vi "Decimate DFD.vi"(8 "error in (no error)":errorcluster, 10 "output fs[Hz]":dbl=6500.0 format="%#_13g", 11 "Waveforms in":waveform(dbl)[](array[waveform])) -> (0 "error out":errorcluster, 3 "waveforms out":waveform(dbl)[](array[waveform]))   [LabVIEW 2019, in "Instrument.Lockin.lvlib" / "Instrument.DAQ.lvclass"]
uses:
  Instrument.DAQ.lvclass
  <vilib>/addons/Digital Filter Design/_Objects.llb/DFD Multirate Filtering Mode.ctl
  <vilib>/Analysis/2dsp.llb/Decimate (single shot, DBL).vi
  <vilib>/addons/Digital Filter Design/NI_DigFilterLicensed.lvlib
  <vilib>/addons/Digital Filter Design/_Objects.llb/DFD Multirate Filter Specification (Design).ctl
  <vilib>/Analysis/NI_AALPro.lvlib
  <vilib>/measure/NI_MAPro.lvlib
  <vilib>/addons/Digital Filter Design/_Objects.llb/DFD Filter Ripple Specification (Design).ctl
  <vilib>/addons/Digital Filter Design/Multirate.llb/DFD MRate Filtering for Single Block (Wfm NChan).vi
  <vilib>/measure/maresamp.llb/Resample N Waveforms (continuous).vi
  <vilib>/addons/Digital Filter Design/Multirate.llb/DFD NStage MRate Filtering for Single Block (Wfm).vi
  <vilib>/addons/Digital Filter Design/Multirate.llb/DFD NStage MRate Filtering (Wfm).vi
panel:
  out "x != y?":bool
  out "x/y":dbl
  out "Magnitude Response":cluster{"f0":dbl, "df":dbl, "values":dbl[]}[](graph)
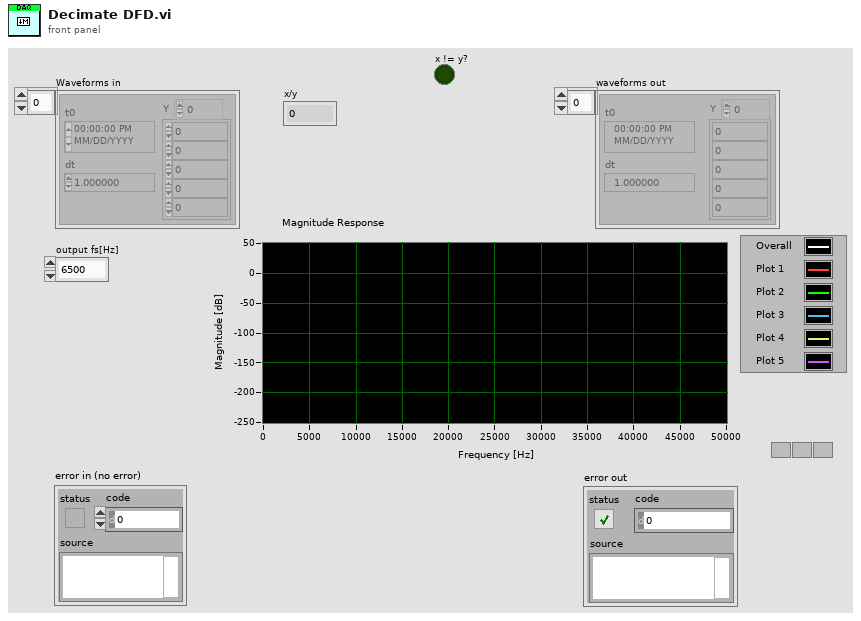
[diagram p1: front panel]
types:
  T1 = typedef "NI_DigFilterLicensed.lvlib/DFD Multirate Filtering Mode.ctl" = u16
  T2 = typedef "NI_DigFilterLicensed.lvlib/DFD Filter Ripple Specification (Design).ctl" = cluster{"passband":dbl, "stopband":dbl, "dB/linear? (T: dB)":bool}
  T3 = typedef "NI_DigFilterLicensed.lvlib/DFD Multirate Filter Specification (Design).ctl" = cluster{"fpass":dbl, "fstop":dbl}
  T4 = typedef "NI_DigFilterLicensed.lvlib/DFD Multirate Filter Obj.ctl" = cluster{"mMRate_Structure":enum16{"CIC", "FIR", "IIR", "Lattice"}, "mMRate_Mode":T5, "mMRate_Factor":i32, "mMRate_FIRParams":cluster{"mMRate_FIR_H":dbl[], "mMRate_FIR_IsNyquist?":bool, "mMRate_FIR_IsSymmetric?":bool}, "mMRate_CICParams":cluster{"mMRate_CIC_#Stage":i32, "mMRate_CIC_Lag":i32, "mMRate_CIC_Type":enum16{"Lowpass", "Highpass"}}, "mMRate_Order":i32, "mMRate_Version":string, "mMRate_Comments":string, "mMRate_RationalFactor":cluster{"mMRate_L":i32, "mMRate_M":i32}, "mMRate_Fs":dbl, "mMRate_Quantized?":bool, "mMRate_QFilterGain":dbl, "mMRate_CoefWl":i16, "mMRate_Scaling":cluster{"mMRate_ScaleByPowerOf2?":bool, "mMRate_ScaleType":T6}, "mMRate_InputWl":i16, "mMRate_OutputWl":i16, "mMRate_OutputMode":T7, "mMRate_MultMode":T8, "mMRate_BitPruning":bool, "mMRate_GainWl":i16, "mMRate_OutputFwl":i16, "mMRate_SumIwl":i16, "mMRate_InputIwl ":i16, "mMRate_SumWl":i16, "mMRate_CoefIwl":i16}
  T5 = typedef "NI_DigFilterLicensed.lvlib/DFD Multirate Mode.ctl" = i16
  T6 = typedef "NI_DigFilterLicensed.lvlib/DFD Coef Norm Type.ctl" = enum16{"No Norm", "Time Domain 1-Norm", "Time Domain 2-Norm", "Time Domain Inf-Norm"}
  T7 = typedef "NI_DigFilterLicensed.lvlib/DFD Round-off Mode.ctl" = enum16{"Nearest", "Truncation"}
  T8 = typedef "NI_DigFilterLicensed.lvlib/DFD FXP MRate Multiply Mode.ctl" = enum16{"Truncated", "Full"}
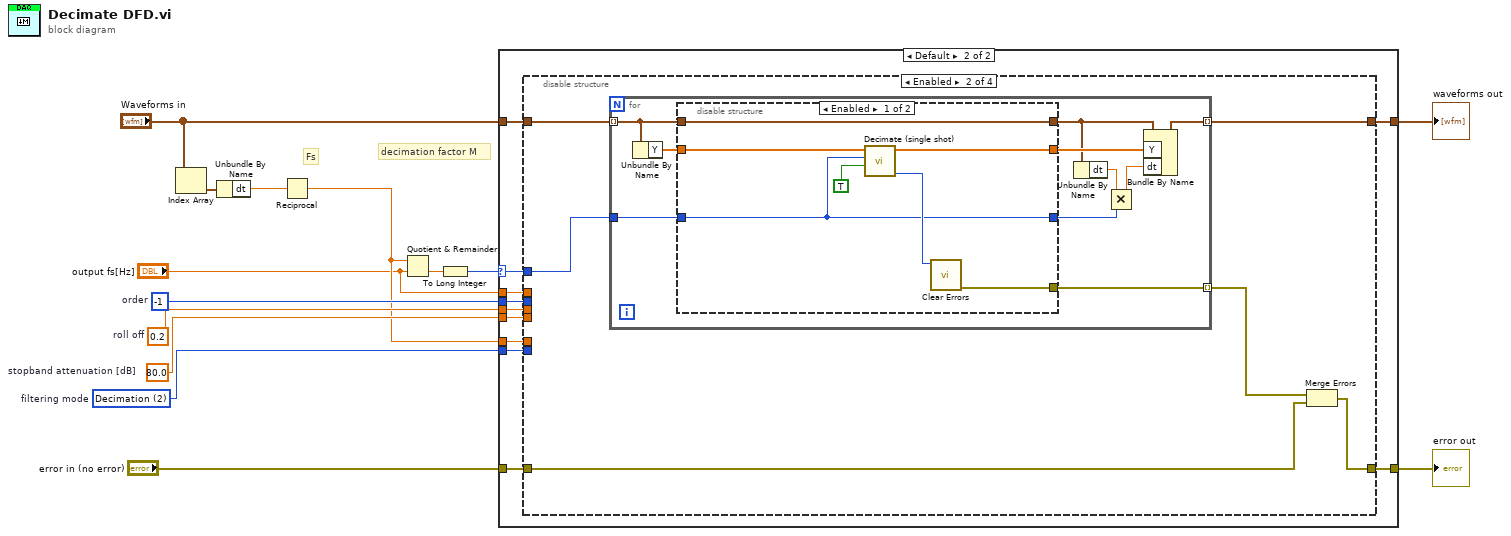
[diagram p0: block diagram]
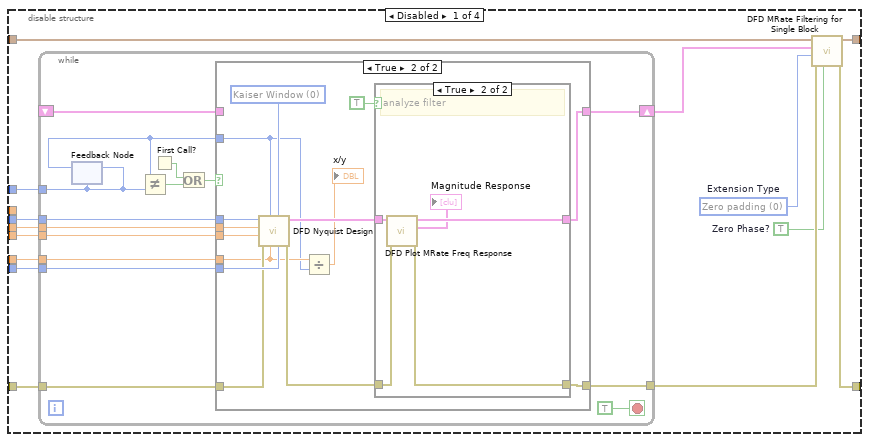
[diagram p3: hidden frame]
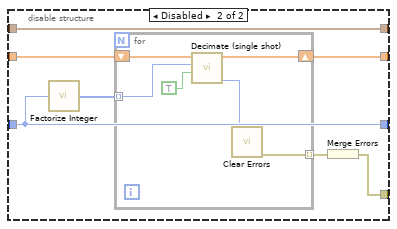
[diagram p6: hidden frame]
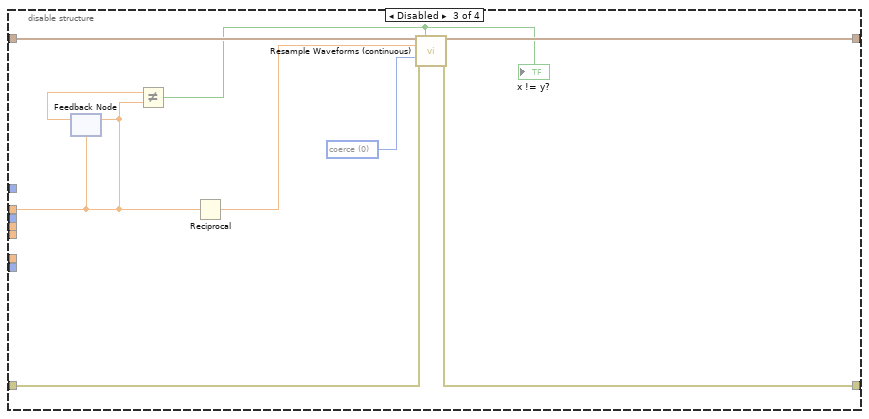
[diagram p7: hidden frame]
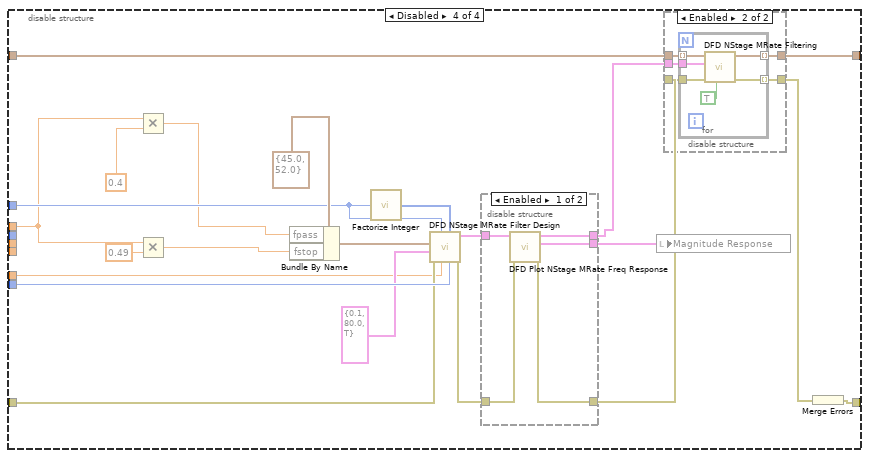
[diagram p8: hidden frame]
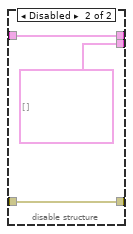
[diagram p9: hidden frame]
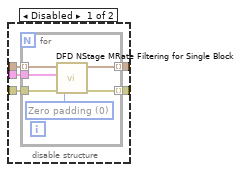
[diagram p10: hidden frame]
diagram:
  w13 = -1  # order
  w10 = 80.0  # stopband attenuation [dB]
  w11 = T1 2 items=["No Rate Change", "Interpolation", "Decimation"]  # filtering mode
  w14 = 0.2  # roll off
  # "Fs"
  # "decimation factor M"
  n1 = Index Array(array="Waveforms in") -> (element=w7:waveform(dbl))  [unwired: 1 in]
  n2 = Unbundle By Name(w7) -> ("dt"=w3:dbl)
  n3 = Reciprocal(x=w3) -> (1/x=w2:dbl)
  n4 = Quotient & Remainder(x=w2, y="output fs[Hz]") -> (floor(x/y)=w12:dbl)  [unwired: 1 out]
  n5 = To Long Integer(number=w12) -> (32bit integer=w8:i32)
  n6 = case shown="Default" w8 {
    selector: w8 -> [_ w21]
    tunnel: w14 -> [_ w27]
    tunnel: w11 -> [_ w26]
    tunnel: w10 -> [_ w25]
    tunnel: w13 -> [_ w24]
    tunnel: "Waveforms in" -> [w16 w20]
    tunnel: [w16 w23] -> w9
    tunnel: w2 -> [_ w22]
    tunnel: "output fs[Hz]" -> [_ w19]
    tunnel: [w15 w18] -> w5
    tunnel: "error in (no error)" -> [w15 w17]
    frame 0, 1 {
    }
    frame Default {
      n7 = disable-structure shown="Enabled" {
        disable-tunnel: w27 -> [w41 _ _ _]
        disable-tunnel: w26 -> [w40 _ _ w145]
        disable-tunnel: w25 -> [w39 _ _ _]
        disable-tunnel: w24 -> [w38 _ _ _]
        disable-tunnel: [w37 w81 w123 w144] -> w23
        disable-tunnel: w22 -> [w36 _ _ w125]
        disable-tunnel: w20 -> [w33 w82 w124 w128]
        disable-tunnel: w21 -> [w32 w85 _ w136]
        disable-tunnel: w19 -> [_ _ w118 w133]
        disable-tunnel: [w31 w83 w121 w137] -> w18
        disable-tunnel: w17 -> [w28 w84 w122 w140]
        frame Disabled {
          w29 = TRUE  # Zero Phase?
          w30 = u16 0 items=["Zero padding", "Symmetric", "Periodic"]  # Extension Type
          n8 = while {
            tunnel: w41 -> [w56]
            tunnel: w40 -> [w55]
            tunnel: w39 -> [w54]
            tunnel: w38 -> [w53]
            tunnel: w36 -> [w52]
            tunnel: [w50] -> w34
            shift-right: [w51] -> w35
            shift-left: _ -> [w48]
            tunnel: w32 -> [w43]
            tunnel: w28 -> [w44]
            stop <- TRUE stop-if-true
            n9 = feedback #1(w43) -> (w42:i32)
            n10 = feedback-in #1(w43) -> ()
            n11 = Not Equal?(x=w42, y=w43) -> (x != y?=w46:bool)
            n12 = First Call?() -> (First Call?: T/F=w47:bool)
            n13 = Or(x=w47, y=w46) -> (x .or. y?=w45:bool)
            n14 = case shown="True" w45 {
              tunnel: w56 -> [_ w72]
              tunnel: w55 -> [_ w71]
              tunnel: w54 -> [_ w70]
              tunnel: w53 -> [_ w69]
              tunnel: w52 -> [_ w61]
              tunnel: [w57 w66] -> w51
              tunnel: [w58 w65] -> w50
              tunnel: w48 -> [w57 _]
              tunnel: w42 -> [_ w60]
              tunnel: w44 -> [w58 w62]
              frame False {
              }
              frame True {
                w68 = u16 0 items=["Kaiser Window", "Dolph-Chebyshev Window", "Equi-Ripple", "Positive Equi-Ripple"] ("method")
                n15 = call <vilib>:"DFD Nyquist Design.vi"("filtering mode"=w71, "method"=w68, "fs in [Hz]"=w61, "factor"=w60, "error in (no error)"=w62, "stopband attenuation [dB]"=w70, "roll off"=w72, "order"=w69) -> ("error out"=w63:errorcluster, "multirate filter out"=w67:T4)  [unwired: 2 out]
                n16 = Divide(x=w61, y=w60) -> (x/y=→"x/y":dbl)
                n17 = case shown="True" TRUE {
                  tunnel: w67 -> [w74 w79]
                  tunnel: w63 -> [w73 w76]
                  tunnel: [w74 w78] -> w66
                  tunnel: [w73 w75] -> w65
                  frame False {
                  }
                  frame True {
                    # "analyze filter"
                    n18 = call <vilib>:"DFD Plot MRate Freq Response.vi"("error in (no error)"=w76, "multirate filter in"=w79) -> ("error out"=w75:errorcluster, "magnitude response"=→"Magnitude Response":cluster{"f0":dbl, "df":dbl, "values":dbl[]}[], "multirate filter out"=w78:T4)  [unwired: 5 in, 2 out]
                  }
                }
              }
            }
          }
          n19 = call-poly <vilib>:"DFD MRate Filtering for Single Block.vi"("zero phase? (T)"=w29, "error in (no error)"=w34, "extension type"=w30, "multirate filter"=w35, "signal in"=w33) -> ("error out"=w31:errorcluster, "signal out"=w37:waveform(dbl)[])  [unwired: 5 out]
        }
        frame Enabled {
          n20 = for {
            tunnel: w82 -> [w94] mode=indexing
            tunnel: [w91] -> w81 mode=indexing
            tunnel: w85 -> [w93]
            tunnel: [w92] -> w80 mode=indexing
            n21 = Unbundle By Name(w94) -> ("Y"=w95:dbl[])
            n22 = disable-structure shown="Enabled" {
              disable-tunnel: w95 -> [w102 w109]
              disable-tunnel: w94 -> [w98 w105]
              disable-tunnel: [w98 w105] -> w89
              disable-tunnel: w93 -> [w96 w103]
              disable-tunnel: [w100 w106] -> w92
              disable-tunnel: [w97 w104] -> w90
              disable-tunnel: [w96 w103] -> w87
              frame Enabled {
                n23 = call-poly <vilib>:"Decimate (single shot).vi"("averaging"=TRUE, "decimating factor"=w96, "X"=w102) -> ("error"=w101:i32, "Decimated Array"=w97:dbl[])  [unwired: 7 in]
                n24 = call <vilib>:"Clear Errors.vi"("specific error code to clear (0: all)"=w101) -> ("error out"=w100:errorcluster)  [unwired: 5 in, 1 out]
              }
              frame Disabled {
                n25 = call "Factorize Integer.vi"("Integer in"=w103) -> ("Integer Factors"=w108:i32[])
                n26 = for {
                  shift-right: [w114] -> w104
                  shift-left: w109 -> [w115]
                  tunnel: w108 -> [w113] mode=indexing
                  tunnel: [w110] -> w107 mode=indexing
                  n27 = call-poly <vilib>:"Decimate (single shot).vi"("averaging"=TRUE, "decimating factor"=w113, "X"=w115) -> ("error"=w111:i32, "Decimated Array"=w114:dbl[])  [unwired: 7 in]
                  n28 = call <vilib>:"Clear Errors.vi"("specific error code to clear (0: all)"=w111) -> ("error out"=w110:errorcluster)  [unwired: 5 in, 1 out]
                }
                n29 = Merge Errors(w107) -> (w106:errorcluster)
              }
            }
            n30 = Unbundle By Name(w89) -> ("dt"=w88:dbl)
            n31 = Multiply(x=w88, y=w87) -> (x*y=w86:dbl)
            n32 = Bundle By Name(cluster=w89, "Y"=w90, "dt"=w86) -> (w91:waveform(dbl))
          }
          n33 = Merge Errors(w80, w84) -> (w83:errorcluster)
        }
        frame Disabled {
          w116 = u16 0 items=["coerce", "linear", "spline", "FIR filter"] ("interpolation mode")
          n34 = feedback #2(w118) -> (w119:dbl)
          n35 = feedback-in #2(w118) -> ()
          n36 = Not Equal?(x=w119, y=w118) -> (x != y?=w117:bool)
          "x != y?" <- w117
          n37 = Reciprocal(x=w118) -> (1/x=w120:dbl)
          n38 = call-poly <vilib>:"Resample Waveforms (continuous).vi"("waveforms in"=w124, "reset"=w117, "dt"=w120, "interpolation mode"=w116, "error in (no error)"=w122) -> ("resampled waveforms out"=w123:waveform(dbl)[], "error out"=w121:errorcluster)  [unwired: 6 in, 3 out]
        }
        frame Disabled {
          n39 = Multiply(x=w133, y=0.4) -> (x*y=w132:dbl)
          n40 = Multiply(x=w133, y=0.49) -> (x*y=w127:dbl)
          n41 = Bundle By Name(cluster=T3 {"fpass"=45.0, "fstop"=52.0} ("freq specs [Hz]"), "fpass"=w132, "fstop"=w127) -> (w141:T3)
          n42 = call "Factorize Integer.vi"("Integer in"=w136) -> ("Integer Factors"=w126:i32[])
          n43 = call <vilib>:"DFD NStage MRate Filter Design.vi"("filtering mode"=w145, "manual factorization"=w126, "fs in [Hz]"=w125, "factor"=w136, "error in (no error)"=w140, "ripple specs"=T2 {"passband"=0.1, "stopband"=80.0, "dB/linear? (T: dB)"=TRUE}, "freq specs [Hz]"=w141) -> ("error out"=w135:errorcluster, "multirate filters out"=w138:T4[])  [unwired: 3 in]
          n44 = disable-structure shown="Enabled" {
            disable-tunnel: [w151 cluster{"f0":dbl, "df":dbl, "values":dbl[]}[] [] ("Magnitude Response")] -> w146
            disable-tunnel: w138 -> [w150 w154]
            disable-tunnel: [w149 w154] -> w129
            disable-tunnel: w135 -> [w148 w153]
            disable-tunnel: [w147 w153] -> w134
            frame Enabled {
              n45 = call <vilib>:"DFD Plot NStage MRate Freq Response.vi"("error in (no error)"=w148, "multirate filters in"=w150) -> ("error out"=w147:errorcluster, "magnitude responses"=w151:cluster{"f0":dbl, "df":dbl, "values":dbl[]}[], "multirate filters out"=w149:T4[])  [unwired: 6 in, 1 out]
            }
            frame Disabled {
            }
          }
          n46 = local write "Magnitude Response"(w146) -> ()
          n47 = disable-structure shown="Enabled" {
            disable-tunnel: [w159 w169] -> w144
            disable-tunnel: [w158 w166] -> w139
            disable-tunnel: w134 -> [w157 w167]
            disable-tunnel: w128 -> [w156 w170]
            disable-tunnel: w129 -> [w155 w168]
            frame Disabled {
              n48 = for {
                tunnel: w156 -> [w165] mode=indexing
                tunnel: w155 -> [w164]
                tunnel: [w163] -> w159 mode=indexing
                tunnel: w157 -> [w161]
                tunnel: [w160] -> w158 mode=indexing
                w162 = u16 0 items=["Zero padding", "Symmetric", "Periodic"] ("extension type")
                n49 = call-poly <vilib>:"DFD NStage MRate Filtering for Single Block.vi"("error in (no error)"=w161, "extension type"=w162, "multirate filters"=w164, "signal in"=w165) -> ("error out"=w160:errorcluster, "signal out"=w163:waveform(dbl))  [unwired: 6 in]
              }
            }
            frame Enabled {
              n50 = for {
                tunnel: w170 -> [w176] mode=indexing
                tunnel: [w175] -> w169 mode=indexing
                tunnel: w168 -> [w174]
                tunnel: w167 -> [w172]
                tunnel: [w171] -> w166 mode=indexing
                n51 = call-poly <vilib>:"DFD NStage MRate Filtering.vi"("zero phase? (T)"=TRUE, "error in (no error)"=w172, "multirate filters"=w174, "signal in"=w176) -> ("error out"=w171:errorcluster, "signal out"=w175:waveform(dbl))  [unwired: 1 in, 5 out]
              }
            }
          }
          n52 = Merge Errors(w139) -> (w137:errorcluster)
        }
      }
    }
  }
  "waveforms out" <- w9
  "error out" <- w5
